vi "Attitude Indicator Init.vi"(3 "Container State":T5={"Indicator?"=TRUE, "Run Mode?"=FALSE, " Refnum"=refnum}, 4 "Previous State":variant=variant(cluster{"Draw Options":cluster{"Text Color":u32, "Wing Color":u32, "Dial Outline Color":u32, "Sky Color":u32, "Ground Color":u32, "Horizon Line Color":u32, "Outline Color":u32, "Dial Background Color":u32, "Draw Wings":bool, "Draw Text":bool, "Font Name":string}} {"Draw Options"={"Text Color"=0, "Wing Color"=16751616, "Dial Outline Color"=13816530, "Sky Color"=3381759, "Ground Color"=8213043, "Horizon Line Color"=16777225, "Outline Color"=0, "Dial Background Color"=5987163, "Draw Wings"=TRUE, "Draw Text"=TRUE, "Font Name"="Helvetica"}}), 5 "Previous Version":T4={"Major"=2, "Minor"=0, "Fix"=0, "Build"=0}) -> (2 "Current State":T1={"Draw Options"={"Text Color"=16777228, "Wing Color"=16751616, "Dial Outline Color"=13816530, "Sky Color"=3381759, "Ground Color"=8213043, "Horizon Line Color"=16777225, "Outline Color"=0, "Dial Background Color"=5987163, "Draw Wings"=TRUE, "Draw Text"=TRUE, "Font Name"="Helvetica", "Angle units"=enum."Radians"}})   [LabVIEW 2017, in "Attitude Indicator.xctl"]
uses:
  <vilib>/robotics/Controls/Attitude Indicator/Attitude Indicator.xctl
  <vilib>/robotics/Controls/Attitude Indicator/_Attitude Indicator Support Files/Attitude Indicator State.ctl
  <vilib>/robotics/Controls/Attitude Indicator/Attitude Picture/Draw Options.ctl
  <vilib>/robotics/Controls/Utilities/Angle Units.ctl
  <vilib>/_xctls/Container State.ctl
  <vilib>/_xctls/Version.ctl
  <vilib>/robotics/Controls/Attitude Indicator/Attitude Picture/NI_Robotics_Attitude Picture.lvlib
  <vilib>/robotics/Controls/Utilities/NI_Robotics_Control Utilities.lvlib
  <vilib>/_xctls/XControlSupport.lvlib
panel:
  in  "Default Indicator State":T1={"Draw Options"={"Text Color"=16777228, "Wing Color"=16751616, "Dial Outline Color"=13816530, "Sky Color"=3381759, "Ground Color"=8213043, "Horizon Line Color"=16777225, "Outline Color"=0, "Dial Background Color"=5987163, "Draw Wings"=TRUE, "Draw Text"=TRUE, "Font Name"="Helvetica", "Angle units"=enum."Degrees"}}
  in  "Default Control State":T1={"Draw Options"={"Text Color"=16777228, "Wing Color"=16751616, "Dial Outline Color"=13816530, "Sky Color"=3381759, "Ground Color"=8213043, "Horizon Line Color"=16777225, "Outline Color"=0, "Dial Background Color"=5987163, "Draw Wings"=TRUE, "Draw Text"=TRUE, "Font Name"="Helvetica", "Angle units"=enum."Degrees"}}
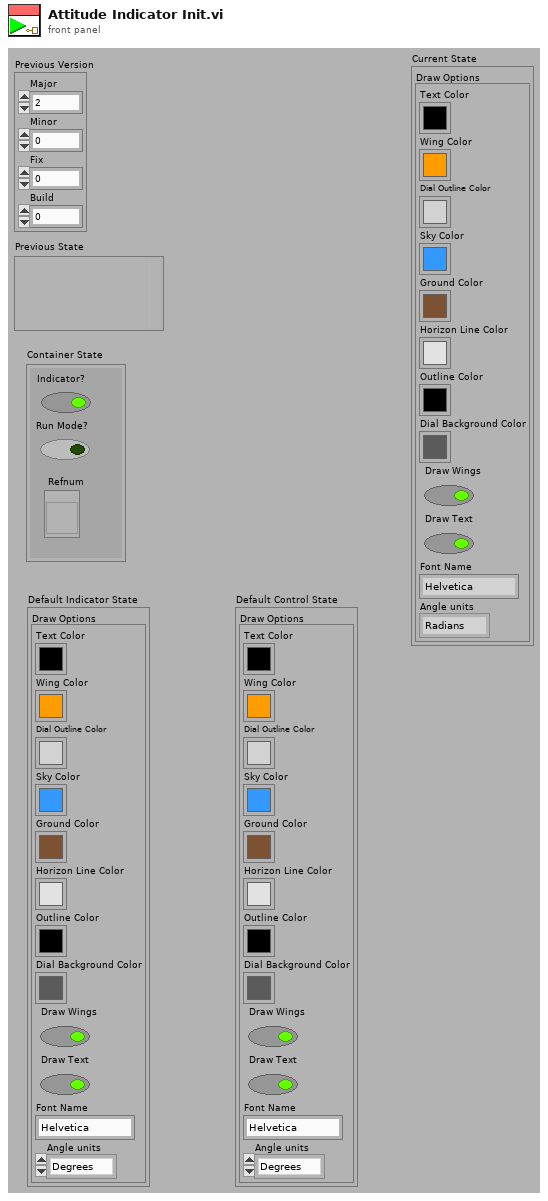
[diagram p1: front panel]
types:
  T1 = typedef "Attitude Indicator.xctl/Attitude Indicator State.ctl" = cluster{"Draw Options":T2}
  T2 = typedef "NI_Robotics_Attitude Picture.lvlib/Draw Options.ctl" = cluster{"Text Color":u32, "Wing Color":u32, "Dial Outline Color":u32, "Sky Color":u32, "Ground Color":u32, "Horizon Line Color":u32, "Outline Color":u32, "Dial Background Color":u32, "Draw Wings":bool, "Draw Text":bool, "Font Name":string, "Angle units":T3}
  T3 = typedef "NI_Robotics_Control Utilities.lvlib/Angle Units.ctl" = enum16{"Radians", "Degrees"}
  T4 = typedef "XControlSupport.lvlib/Version.ctl" = cluster{"Major":u16, "Minor":u16, "Fix":u16, "Build":u16}
  T5 = typedef "XControlSupport.lvlib/Container State.ctl" = cluster{"Indicator?":bool, "Run Mode?":bool, " Refnum":refnum<vi>}
  T6 = cluster{"Text Color":u32, "Wing Color":u32, "Dial Outline Color":u32, "Sky Color":u32, "Ground Color":u32, "Horizon Line Color":u32, "Outline Color":u32, "Dial Background Color":u32, "Font Name:":string, "Draw Wings?":bool, "Draw Text?":bool}
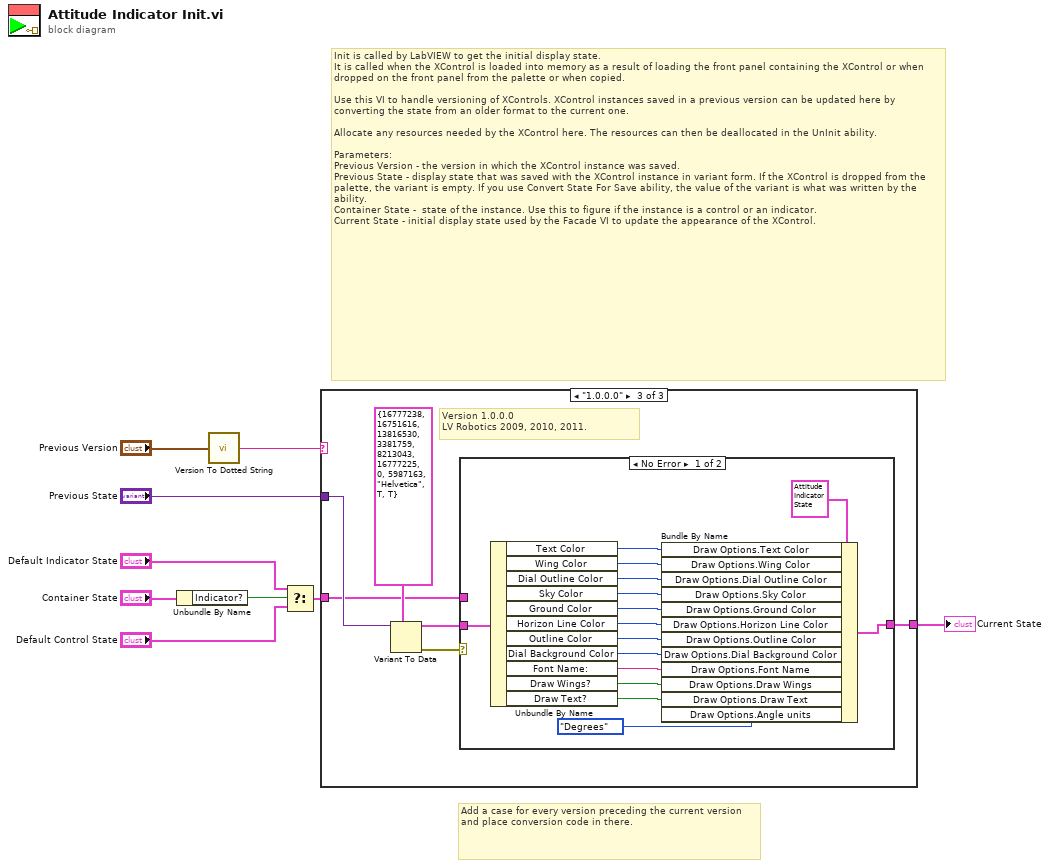
[diagram p0: block diagram]
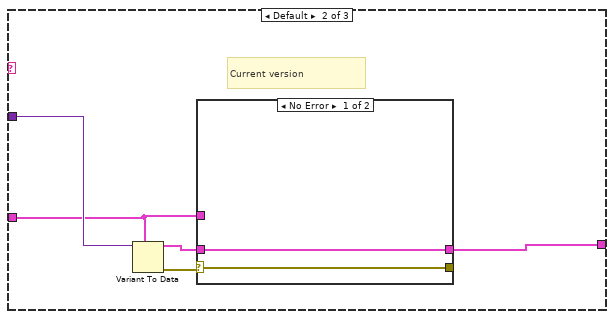
[diagram p3: hidden frame]
diagram:
  # "Add a case for every version preceding the current version and place conversion code in there."
  # "Init is called by LabVIEW to get the initial display state.\nIt is called when the XControl is loaded into memory as a result of loading the front panel containing the XControl or when dropped on the front panel from the palette or when copied.\n\nUse this VI to handle versioning of XControls. XControl instances saved in a previous version can be updated here by converting the state from an older format to the current one.\n\nAllocate any resources needed by the XControl here. The resources can then be deallocated in the UnInit ability.\n\nParameters:\nPrevious Version - the version in which the XControl instance was saved.\nPrevious State - display state that was saved with the XControl instance in variant form. If the XControl is dropped from the palette, the variant is empty. If you use Convert State For Save ability, the value of the variant is what was written by the ability. \nContainer State -  state of the instance. Use this to figure if the instance is a control or an indicator.\nCurrent State - initial display state used by the Facade VI to update the appearance of the XControl."
  n1 = Unbundle By Name("Container State") -> ("Indicator?"=w4:bool)
  n2 = call <vilib>:"Version To Dotted String.vi"("Version"="Previous Version") -> ("String Version"=w1:string)
  n3 = Select(t="Default Indicator State", s=w4, f="Default Control State") -> (s? t:f=w3:T1)
  n4 = case shown="\"1.0.0.0\"" w1 {
    tunnel: "Previous State" -> [_ w15 w25]
    tunnel: [w10 w11 w22] -> w8
    tunnel: w3 -> [w10 w12 w20]
    frame "0.0.0.0" {
      # "Just created, use default state"
    }
    frame Default {
      # "Current version"
      n5 = Variant To Data(type=w12, Variant=w15) -> (data=w13:T1, error out=w14:errorcluster)  [unwired: 1 in]
      n6 = case shown="No Error" w14 {
        selector: w14 -> [w17 w18]
        tunnel: w13 -> [w16 _]
        tunnel: [w16 w19] -> w11
        tunnel: w12 -> [_ w19]
        tunnel: [w17 w18] -> _
        frame No Error {
        }
        frame Error {
          # "Error converting previously \nsaved state. Use default instead."
        }
      }
    }
    frame "1.0.0.0" {
      # "Version 1.0.0.0\nLV Robotics 2009, 2010, 2011."
      n7 = Variant To Data(type=T6 {"Text Color"=16777238, "Wing Color"=16751616, "Dial Outline Color"=13816530, "Sky Color"=3381759, "Ground Color"=8213043, "Horizon Line Color"=16777225, "Outline Color"=0, "Dial Background Color"=5987163, "Font Name:"="Helvetica", "Draw Wings?"=TRUE, "Draw Text?"=TRUE} ("1.0.0.0 State"), Variant=w25) -> (data=w23:T6, error out=w24:errorcluster)  [unwired: 1 in]
      n8 = case shown="No Error" w24 {
        tunnel: w23 -> [w40 _]
        tunnel: [w28 w41] -> w22
        tunnel: w20 -> [_ w41]
        frame No Error {
          n9 = Unbundle By Name(w40) -> ("Text Color"=w29:u32, "Wing Color"=w30:u32, "Dial Outline Color"=w31:u32, "Sky Color"=w32:u32, "Ground Color"=w33:u32, "Horizon Line Color"=w34:u32, "Outline Color"=w35:u32, "Dial Background Color"=w36:u32, "Font Name:"=w37:string, "Draw Wings?"=w38:bool, "Draw Text?"=w39:bool)
          n10 = Bundle By Name(cluster=T1 {"Draw Options"={"Text Color"=0, "Wing Color"=0, "Dial Outline Color"=0, "Sky Color"=0, "Ground Color"=0, "Horizon Line Color"=0, "Outline Color"=0, "Dial Background Color"=0, "Draw Wings"=FALSE, "Draw Text"=FALSE, "Font Name"="", "Angle units"=enum."Degrees"}} ("State"), "Draw Options.Text Color"=w29, "Draw Options.Wing Color"=w30, "Draw Options.Dial Outline Color"=w31, "Draw Options.Sky Color"=w32, "Draw Options.Ground Color"=w33, "Draw Options.Horizon Line Color"=w34, "Draw Options.Outline Color"=w35, "Draw Options.Dial Background Color"=w36, "Draw Options.Font Name"=w37, "Draw Options.Draw Wings"=w38, "Draw Options.Draw Text"=w39, "Draw Options.Angle units"=Angle_Units."Degrees") -> (w28:T1)
        }
        frame Error {
          # "Error converting previously \nsaved state. Use default instead."
        }
      }
    }
  }
  "Current State" <- w8
